vi "Overlay X-Center Line.vi"(6 "Color":u32(colorbox)=16711680, 8 "error in":errorcluster, 11 "Image Dst Out":T1) -> (0 "error out":errorcluster, 3 "Image Out":T1)   [LabVIEW 2013]
doc: "Overlays a center line in the middle of an image."
uses:
  <vilib>/vision/Image Controls.llb/IMAQ Image.ctl
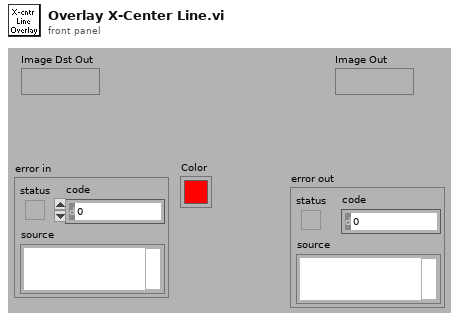
[diagram p1: front panel]
types:
  T1 = typedef "IMAQ Image.ctl" = refnum<image>
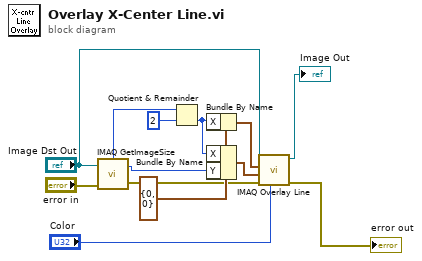
[diagram p0: block diagram]
diagram:
  w9 = cluster{"X":i32, "Y":i32} {"X"=0, "Y"=0} ("Start Point")
  n1 = call "IMAQ GetImageSize"("Image"="Image Dst Out", "error in (no error)"="error in") -> ("Y Resolution"=w11:i32, "X Resolution"=w2:i32, "error out"=w4:errorcluster)  [unwired: 2 out]
  n2 = Quotient & Remainder(x=w2, y=2) -> (floor(x/y)=w10:i32)  [unwired: 1 out]
  n3 = Bundle By Name(cluster=w9, "X"=w10) -> (w7:cluster{"X":i32, "Y":i32})
  n4 = Bundle By Name(cluster=w9, "X"=w10, "Y"=w11) -> (w8:cluster{"X":i32, "Y":i32})
  n5 = call "IMAQ Overlay Line"("Color"="Color", "error in (no error)"=w4, "End Point"=w8, "Start Point"=w7, "Image"="Image Dst Out") -> ("error out"=→"error out":errorcluster, "Image Out"=→"Image Out":T1)  [unwired: 1 in, 4 out]
